vi "Increment Context I32.vi"(8 "error in (no error)":errorcluster, 11 "Context in":refnum<class "Context.lvclass">) -> (0 "error out":errorcluster, 3 "Context out":refnum<class "Context.lvclass">)   [LabVIEW 2021, in "Context.lvlib" / "Context.lvclass"]
uses:
  Context.lvclass
  Context.lvclass/Context.ctl
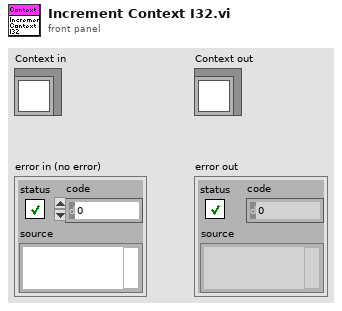
[diagram p1: front panel]
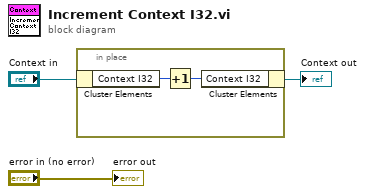
[diagram p0: block diagram]
diagram:
  n1 = in-place {
    n2 = in-place-cluster #1("Context in") -> ("Context I32"=w5:i32)
    n3 = Increment(x=w5) -> (x+1=w4:i32)
    n4 = in-place-cluster #1("Context I32"=w4) -> (→"Context out":refnum<class "Context.lvclass">)
  }
  "error out" <- "error in (no error)"
